vi "DL_Lock_Unlock.vi"(8 "entrée d'erreur (pas d'erreur)":errorcluster, 10 "Control-Client old entrée":refnum<class "Control-Client.lvclass">, 11 "Control-Client new entrée":refnum<class "Control-Client.lvclass">) -> (0 "sortie d'erreur":errorcluster)   [LabVIEW 2015, in "Control-Client.lvclass"]
uses:
  Control-Client.lvclass
  Control-Client.lvclass/Control-Client.ctl
  dependecies/XControls/CellsDL/ControlDL.xctl
  controls/Gauge_pump/Gauge_pump.xctl
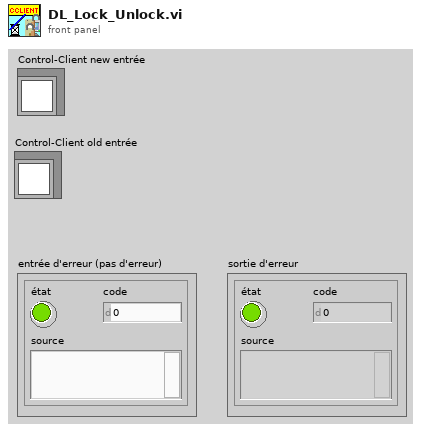
[diagram p1: front panel]
types:
  T1 = enum8{"Enabled", "Disabled", "Disabled and Grayed Out"}
  T2 = typedef "Control-Client.lvclass/Controls-with-permissions_CLIENT.ctl" = cluster{"Server ON/OFF":refnum<vi>, "Detector connect":refnum<vi>, "DL connect":refnum<vi>, "DAQmx connect":refnum<vi>, "All connect":refnum<vi>, "Start measurement":refnum<vi>, "Move Crystal":refnum<vi>, "Relay key heater":refnum<vi>, "Laser Shutter":refnum<vi>, "Accelerator Shutter":refnum<vi>, "Power":refnum<vi>, "Unlock":refnum<vi>, "RT":refnum<vi>, "Faraday Cup":refnum<vi>, "Osc connect":refnum<vi>, "ELYSE pulses":refnum<vi>, "Cells":refnum<vi>, "ControlDL":refnum<vi>, "Pump":refnum<vi>, "# par point":refnum<vi>, "Alarm":refnum<vi>, "oscilloscopeRead":refnum<vi>, "WCM_state":refnum<vi>}
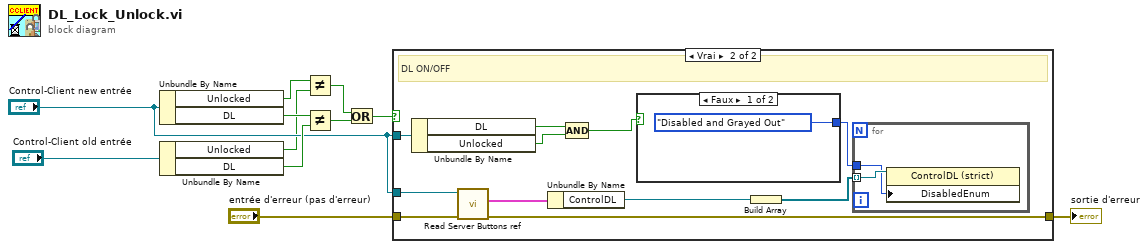
[diagram p0: block diagram]
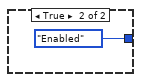
[diagram p3: hidden frame]
diagram:
  n1 = Unbundle By Name("Control-Client new entrée") -> ("Unlocked"=w2:bool, "DL"=w7:bool)
  n2 = Unbundle By Name("Control-Client old entrée") -> ("Unlocked"=w1:bool, "DL"=w8:bool)
  n3 = Not Equal?(x=w2, y=w1) -> (x != y?=w3:bool)
  n4 = Not Equal?(x=w7, y=w8) -> (x != y?=w4:bool)
  n5 = Or(x=w3, y=w4) -> (x .or. y?=w5:bool)
  n6 = case shown="Vrai" w5 {
    tunnel: "Control-Client new entrée" -> [_ w23]
    tunnel: "entrée d'erreur (pas d'erreur)" -> [w12 w22]
    tunnel: [w12 w17] -> w10
    tunnel: "Control-Client new entrée" -> [_ w15]
    frame False {
    }
    frame True {
      # "DL ON/OFF"
      n7 = Unbundle By Name(w15) -> ("DL"=w13:bool, "Unlocked"=w14:bool)
      n8 = call "Read Server Buttons ref.vi"("error in (no error)"=w22, "Control-Client in"=w23) -> ("error out"=w17:errorcluster, "Server Buttons ref"=w21:T2)  [unwired: 7 in, 1 out]
      n9 = Unbundle By Name(w21) -> ("ControlDL"=w20:refnum<vi>)
      n10 = Compound Arithmetic op=AND(w13, w14) -> (w16:bool)
      n11 = case shown="Faux" w16 {
        tunnel: [T1."Disabled and Grayed Out" ("Désactivé") T1."Enabled" ("Désactivé")] -> w19
        frame False {
        }
        frame True {
        }
      }
      n12 = Build Array(w20) -> (w18:refnum<vi>[])
      n13 = for {
        tunnel: w18 -> [w27] mode=indexing
        tunnel: w19 -> [w26]
        n14 = property class="ControlDL (strict)"(reference=w27, "DisabledEnum"=w26) -> ()  [unwired: 1 in, 2 out]
      }
    }
  }
  "sortie d'erreur" <- w10
